vi "Save_Time_Global.vi"() -> ()   [LabVIEW 2018]
panel:
  out "Last Save Time Stamp":timestamp
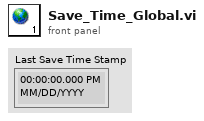
[diagram p1: front panel]
diagram:
